vi "Trial Timestamp Into DB.vi"(8 "error in (no error)":errorcluster, 11 "MatlabExperiment in":refnum<class "MatlabExperiment.lvclass">) -> (0 "error out":errorcluster, 3 "MatlabExperiment out":refnum<class "MatlabExperiment.lvclass">)   [LabVIEW 2014, in "AcquisitionCoreObjects.lvlib" / "MatlabExperiment.lvclass"]
uses:
  MatlabExperiment.lvclass
  Acquisition/Database/StimulationPrimary.ctl
  Acquisition/AcquistionObject/AcquistionObject.lvclass
panel:
  in  "time":timestamp
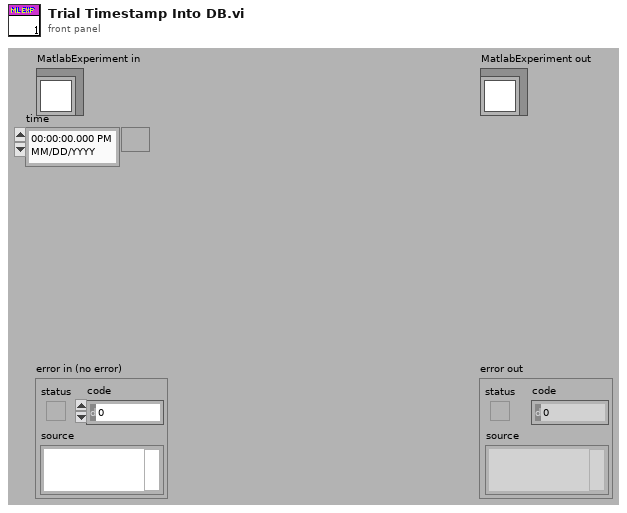
[diagram p1: front panel]
types:
  T1 = cluster{"setup":u8, "session_start_time":u64, "stim_start_time":u64, "time":u64}
  T2 = typedef "NI_Database_API.lvlib/Conn ObjectReference.ctl" = refnum<k1>
  T3 = typedef "StimulationPrimary.ctl" = cluster{"setup":u8, "subject_id":i32, "session_start_time":dbl, "stim_start_time":dbl}
  T4 = cluster{"reference":T2, "table":string, "columns":string[], i32}
  T5 = cluster{cluster{"reference":T2, "table":string, "columns":string[], i32}, "Variant":variant}
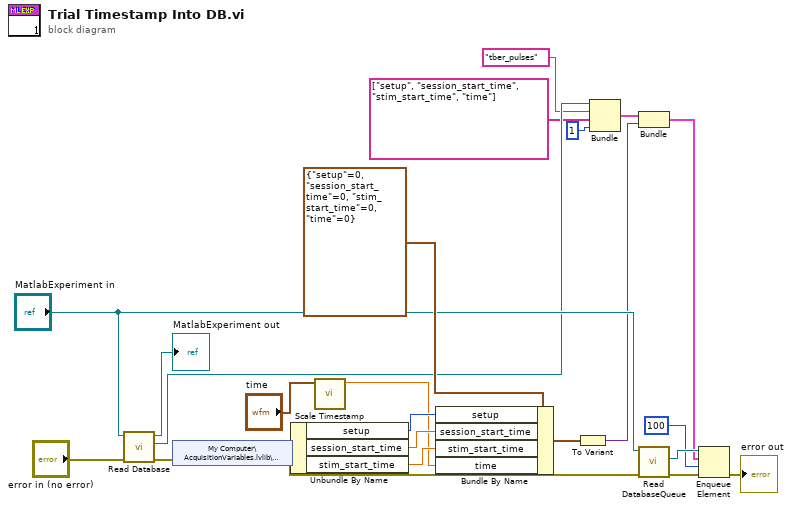
[diagram p0: block diagram]
diagram:
  n1 = call-dynamic "Read Database.vi"("error in (no error)"="error in (no error)", "AcquistionObject in"="MatlabExperiment in") -> ("error out"=w20:errorcluster, "reference"=w13:T2, "AcquistionObject out"=→"MatlabExperiment out":refnum<class "MatlabExperiment.lvclass">)  [unwired: 7 in]
  n2 = shared-variable "My Computer\\AcquisitionVariables.lvlib\\StimulationPK"(error in=w20) -> (w22:T3, error out=w9:errorcluster)
  n3 = Unbundle By Name(w22) -> ("setup"=w24:u8, "session_start_time"=w23:dbl, "stim_start_time"=w19:dbl)
  n4 = call "Scale Timestamp.vi"("Time Stamp"="time") -> ("Scaled timestamp"=w16:dbl)  [unwired: 10 in]
  n5 = Bundle By Name(cluster=T1 {"setup"=0, "session_start_time"=0, "stim_start_time"=0, "time"=0} ("Cluster"), "setup"=w24, "session_start_time"=w23, "stim_start_time"=w19, "time"=w16) -> (w5:T1)
  n6 = To Variant(anything=w5) -> (Variant=w2:variant)
  n7 = Bundle("reference"=w13, "table"="tber_pulses", "columns"=string[] ["setup", "session_start_time", "stim_start_time", "time"], 1) -> (w3:T4)  [unwired: 1 in]
  n8 = Bundle(w3, "Variant"=w2) -> (w1:T5)  [unwired: 1 in]
  n9 = call-dynamic "Read DatabaseQueue.vi"("error in (no error)"=w9, "AcquistionObject in"="MatlabExperiment in") -> ("error out"=w8:errorcluster, "DatabaseQueue"=w10:refnum<queue>)  [unwired: 7 in, 1 out]
  n10 = Enqueue Element(queue=w10, element=w1, timeout in ms (-1)=100, error in (no error)=w8) -> (error out=→"error out":errorcluster)  [unwired: 2 out]
